vi "Volume Desriptor Set Ref.vi"(8 "error in (no error)":errorcluster, 11 "VolumeDescriptor":refnum<k24>) -> (0 "error out":errorcluster, 3 "VGS_VolumeDescriptor out":refnum<class "VGS_VolumeDescriptor.lvclass">)   [LabVIEW 2022 SP3, in "LV_VGS.lvlib" / "VGS_VolumeDescriptor.lvclass"]
uses:
  VGS_VolumeDescriptor.lvclass
  C:/Users/Andrey/Documents/GitHub/LV_VGS/vgs_project.dll
  vgs_project.dll
  VGS_VolumeDescriptor.lvclass/VGS_VolumeDescriptor.ctl
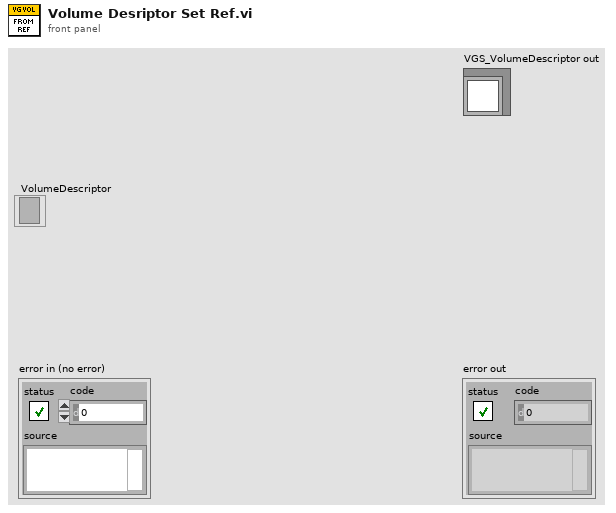
[diagram p1: front panel]
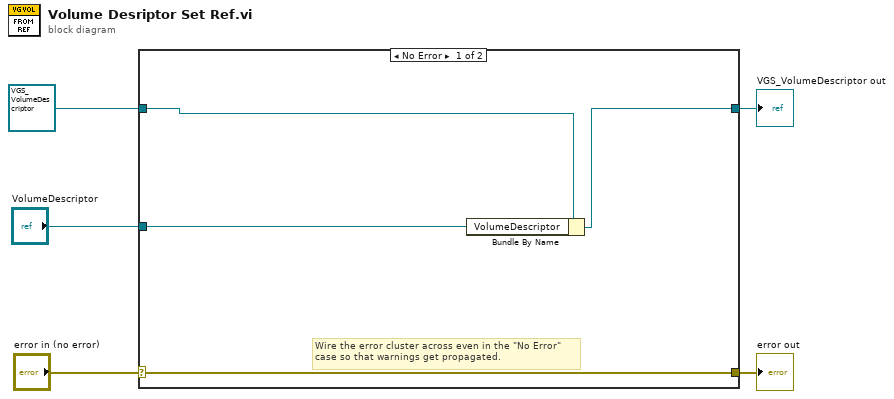
[diagram p0: block diagram]
diagram:
  n1 = case shown="No Error" "error in (no error)" {
    selector: "error in (no error)" -> [w9 w11]
    tunnel: [w9 w11] -> w4
    tunnel: [w6 w10] -> w2
    tunnel: refnum<class "VGS_VolumeDescriptor.lvclass"> refnum ("VGS_VolumeDescriptor in") -> [w8 w10]
    tunnel: "VolumeDescriptor" -> [w7 _]
    frame No Error {
      # "Wire the error cluster across even in the \"No Error\"\ncase so that warnings get propagated."
      n2 = Bundle By Name(cluster=w8, "VolumeDescriptor"=w7) -> (w6:refnum<class "VGS_VolumeDescriptor.lvclass">)
    }
    frame Error {
    }
  }
  "error out" <- w4
  "VGS_VolumeDescriptor out" <- w2
